vi "send refresh.vi"(11 "refresh UI":T1) -> ()   [LabVIEW 2013, in "PL Framework Configuration Tool.lvlib" / "EngineTags.lvclass"]
uses:
  EngineTags.lvclass
  <vilib>/NI/Configuration Framework/Node/RefreshUIEvent.ctl
  <vilib>/NI/Configuration Framework/Node/NISE_CEF_Node.lvclass
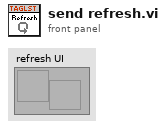
[diagram p1: front panel]
types:
  T1 = typedef "NISE_CEF_Node.lvclass/RefreshUIEvent.ctl" = refnum<user-event>
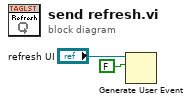
[diagram p0: block diagram]
diagram:
  n1 = Generate User Event(user event="refresh UI", event data cluster=FALSE ("event data")) -> ()  [unwired: 2 in, 2 out]
